vi "Refresh UI.vi"(7 "ComboBox in":refnum<vi>, 9 "Sequences":string, 11 "References":T1) -> (0 "error out":errorcluster, 1 "Standard Sequence":string[][](array[string]), 2 "String":string)   [LabVIEW 2015, in "Sequencer Module editor node.lvclass"]
uses:
  Sequencer Module editor node.lvclass
  <vilib>/NI/DCAF/Tag Editor Core/Table API/Table Manager/object ref.ctl
  <vilib>/NI/DCAF/Tag Editor Core/Configuration Editor/Classes/Engine Parent/Engine Parent Editor Node.lvclass
  <vilib>/NI/DCAF/Tag Editor Core/Configuration Editor/Classes/Module editor node/module editor node.lvclass
  module/configuration/Sequencer Module configuration.lvclass
  module/configuration/Sequencer Module configuration.lvclass/Sequencer Module configuration.ctl
  classes/Sequence/Config/Sequence Config.lvclass
  <vilib>/NI/DCAF/Tag Editor Core/Table API/Table Manager/Table Manager.lvclass
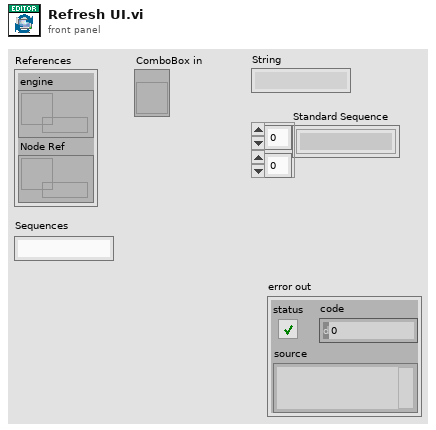
[diagram p1: front panel]
types:
  T1 = typedef "Table Manager.lvlib/Table Manager.lvclass/object ref.ctl" = cluster{"engine":refnum<data-value>, "Node Ref":refnum<data-value>}
  T2 = typedef "Sequencer Module configuration.lvclass/Line.ctl" = cluster{"Sequence":refnum<class "Sequence Config.lvclass">}
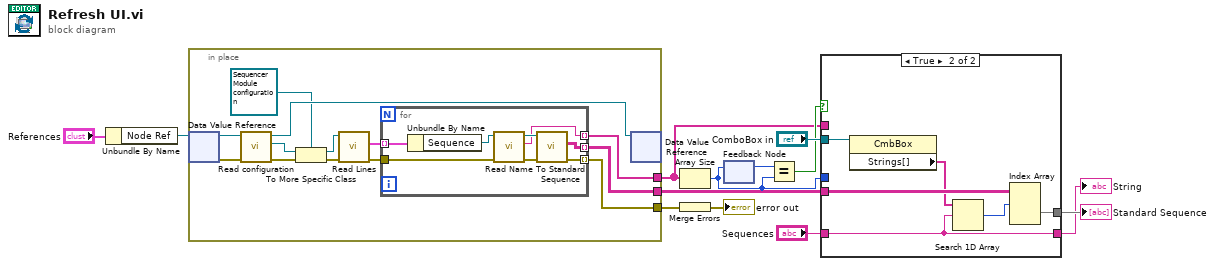
[diagram p0: block diagram]
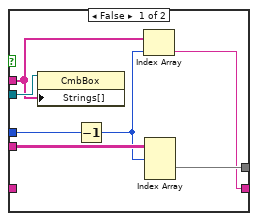
[diagram p2: hidden frame]
diagram:
  n1 = Unbundle By Name("References") -> ("Node Ref"=w13:refnum<data-value>)
  n2 = in-place {
    in-place-border: [w19] -> w12
    in-place-border: [w18] -> w10
    in-place-border: [w14] -> w1
    n3 = in-place-dvr #1(w13) -> (w26:refnum<class "module editor node.lvclass">, w25:errorcluster)
    n4 = call-dynamic "Read configuration.vi"("error in"=w25, "NISE_CEF_serializable node in"=w26) -> ("error out"=w15:errorcluster, "configuration"=w23:refnum<class "NISE_CEF_serializable configuration.lvclass">, "NISE_CEF_serializable node out"=w24:refnum<class "module editor node.lvclass">)  [unwired: 7 in]
    n5 = To More Specific Class(target class=refnum<class "Sequencer Module configuration.lvclass"> refnum ("Sequencer Module configuration"), reference=w23, error in=w15) -> (specific class reference=w21:refnum<class "Sequencer Module configuration.lvclass">, error out=w16:errorcluster)
    n6 = call "Read Lines.vi"("error in (no error)"=w16, "Sequencer Module configuration in"=w21) -> ("error out"=w17:errorcluster, "Lines"=w20:T2[])  [unwired: 7 in, 1 out]
    n7 = for {
      tunnel: w20 -> [w34] mode=indexing
      tunnel: [w31] -> w14 mode=indexing
      tunnel: [w30] -> w19 mode=indexing
      tunnel: [w28] -> w18 mode=indexing
      tunnel: w17 -> [w27]
      n8 = Unbundle By Name(w34) -> ("Sequence"=w33:refnum<class "Sequence Config.lvclass">)
      n9 = call-dynamic "Read Name.vi"("error in (no error)"=w27, "Sequence in"=w33) -> ("error out"=w29:errorcluster, "Name"=w31:string, "Sequence out"=w32:refnum<class "Sequence Config.lvclass">)  [unwired: 7 in]
      n10 = call-dynamic "To Standard Sequence.vi"("error in (no error)"=w29, "Sequence Config in"=w32) -> ("error out"=w28:errorcluster, "Standard Sequence"=w30:string[][])  [unwired: 7 in, 1 out]
    }
    n11 = in-place-dvr #1(w24) -> ()  [unwired: 2 out]
  }
  n12 = Array Size(array=w1) -> (size(s)=w4:i32)
  n13 = Merge Errors(w10) -> (→"error out":errorcluster)
  n14 = feedback-in #2(w4) -> ()
  n15 = feedback #2() -> (w5:i32)  [unwired: 1 in]
  n16 = Equal?(x=w5, y=w4) -> (x = y?=w3:bool)
  n17 = case shown="True" w3 {
    tunnel: w12 -> [w41 w47]
    tunnel: [w40 w46] -> w11
    tunnel: "ComboBox in" -> [w39 w45]
    tunnel: [w36 w43] -> w6
    tunnel: w4 -> [w37 _]
    tunnel: "Sequences" -> [_ w43]
    tunnel: w1 -> [w35 _]
    frame False {
      n18 = property class="CmbBox"(reference=w39, "Strings[]"=w35) -> ()  [unwired: 1 in, 2 out]
      n19 = Decrement(x=w37) -> (x-1=w38:i32)
      n20 = Index Array(array=w35, index=w38) -> (element=w36:string)
      n21 = Index Array(array=w41, index (dim 0)=w38) -> (element=w40:string[][])  [unwired: 2 in]
    }
    frame True {
      n22 = property class="CmbBox"(reference=w45) -> ("Strings[]"=w44:string[])  [unwired: 1 in, 2 out]
      n23 = Search 1D Array(1D array=w44, element=w43) -> (index of element=w42:i32)  [unwired: 1 in]
      n24 = Index Array(array=w47, index (dim 0)=w42) -> (element=w46:string[][])  [unwired: 2 in]
    }
  }
  "String" <- w6
  "Standard Sequence" <- w11
